vi "ITA to II.vi"(11 "Items to Analyze":cluster{"Item Path":path, "Removed?":bool}[](array[cluster])) -> (3 "Item Info":T1[](array[typedef]))   [LabVIEW 2020]
uses:
  <vilib>/addons/analyzer/_vianuishared.llb/VIAnUI Item Info.ctl
  <vilib>/addons/analyzer/_vianuishared.llb/VIAnUI Path Type.ctl
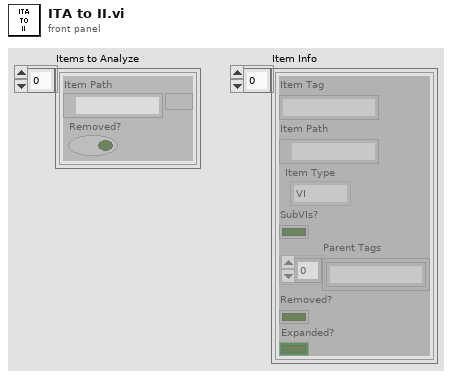
[diagram p1: front panel]
types:
  T1 = typedef "VIAnUI Item Info.ctl" = cluster{"Item Tag":string, "Item Path":path, "Item Type":T2, "SubVIs?":bool, "Parent Tags":string[], "Removed?":bool, "Expanded?":bool}
  T2 = typedef "VIAnUI Path Type.ctl" = enum16{"VI", "LLB", "Folder", "Invalid", "ProjItem"}
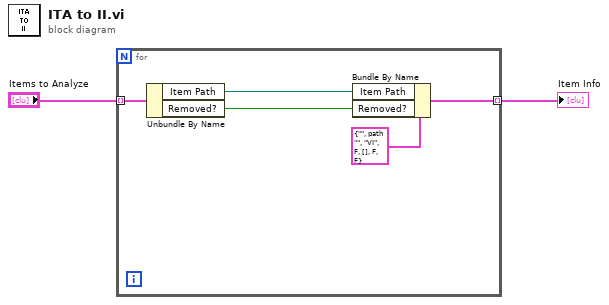
[diagram p0: block diagram]
diagram:
  n1 = for {
    tunnel: "Items to Analyze" -> [w7] mode=indexing
    tunnel: [w3] -> w2 mode=indexing
    n2 = Unbundle By Name(w7) -> ("Item Path"=w5:path, "Removed?"=w4:bool)
    n3 = Bundle By Name(cluster=T1 {"Item Tag"="", "Item Path"=path "", "Item Type"=enum."VI", "SubVIs?"=FALSE, "Parent Tags"=[], "Removed?"=FALSE, "Expanded?"=FALSE} ("Item Info"), "Item Path"=w5, "Removed?"=w4) -> (w3:T1)
  }
  "Item Info" <- w2
